vi "Servo-Motor_Test.vi"() -> ()   [LabVIEW 2019]
panel:
  in  "伺服馬達二角位":tag="A/PWM0"
  in  "伺服馬達一角位":tag="B/PWM2"
  in  "馬達二":dbl(knob) scale=0.0..180.0
  in  "馬達一":dbl(knob) scale=0.0..180.0
  out "Error Out":errorcluster
  in  "Error In":errorcluster
  in  "Stop":bool
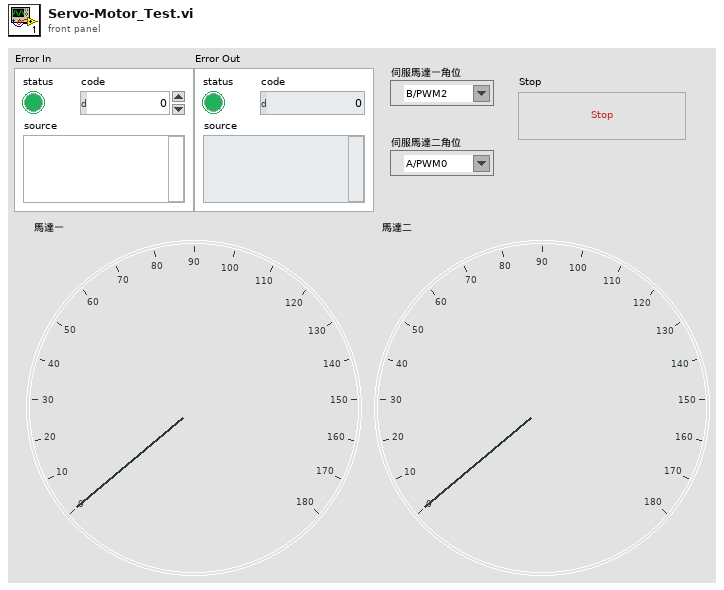
[diagram p1: front panel]
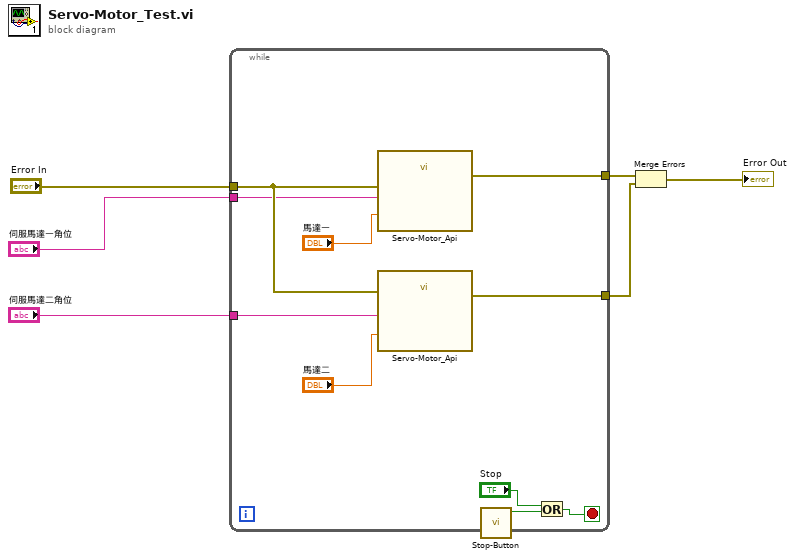
[diagram p0: block diagram]
diagram:
  n1 = while {
    tunnel: "Error In" -> [w13]
    tunnel: [w12] -> w3
    tunnel: "伺服馬達一角位" -> [w11]
    tunnel: "伺服馬達二角位" -> [w10]
    tunnel: [w9] -> w2
    stop <- w16 stop-if-true
    n2 = call "Servo-Motor_Api.vi"("角度"="馬達一", "Error In"=w13, "伺服馬達角位"=w11) -> ("Error Out"=w12:errorcluster)  [unwired: 8 in]
    n3 = call "Servo-Motor_Api.vi"("角度"="馬達二", "Error In"=w13, "伺服馬達角位"=w10) -> ("Error Out"=w9:errorcluster)  [unwired: 8 in]
    n4 = call "Stop-Button.vi"() -> ("顯示按下?"=w14:bool)  [unwired: 10 in, 1 out]
    n5 = Or(x="Stop", y=w14) -> (x .or. y?=w16:bool)
  }
  n6 = Merge Errors(w3, w2) -> (→"Error Out":errorcluster)
